vi "Library_Steering_init.vi"(8 "error in (no error)":errorcluster) -> (0 "error out":errorcluster)   [LabVIEW 2013]
uses:
  My Computer/Controls/Steering Inputs.ctl
  My Computer/Controls/Intuitive Steering.ctl
  My Computer/Controls/Servo Position.ctl
  My Computer/Controls/Fin Arrangement.ctl
  My Computer/Controls/Fin Status.ctl
  My Computer/Controls/Steering Mode.ctl
  My Computer/Controls/Individual Steering.ctl
  My Computer/Controls/IndividualSteering_f(x)_enum.ctl
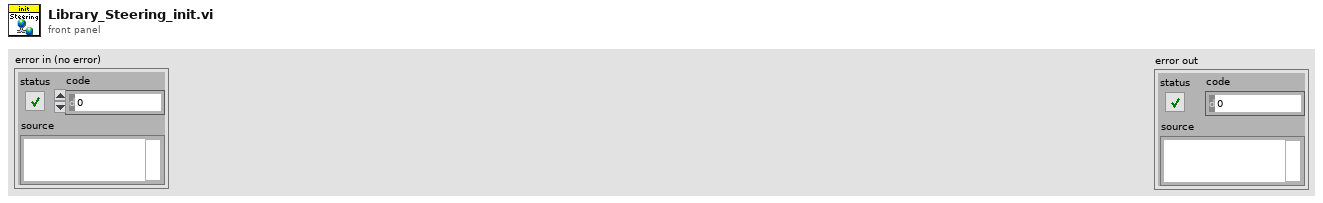
[diagram p1: front panel]
types:
  T1 = typedef "IndividualSteering_f(x)_enum.ctl" = enum16{"sin(x)", "cuttlefish sine", "cuttlefish triangle", "triangle"}
  T2 = typedef "Individual Steering.ctl" = cluster{"Fin Parameters":cluster{"Amplitude":dbl, "Phase Shift":dbl, "Zero Position":dbl}[], "Frequency\n& Direction":dbl, "General A, PS, ZP":cluster{"Amplitude":dbl, "Phase Shift":dbl, "Zero Position":dbl}}[]
  T3 = typedef "Steering Mode.ctl" = enum16{"Intuitive Steering", "Control Allocation", "Individually"}
  T4 = typedef "Intuitive Steering.ctl" = cluster{"Frequency (Hz):":dbl, "Max. Amplitude (°):":dbl, "Phase Shift (/Pi):":dbl, "Flap (°):":dbl, "Flap Saturation:":dbl}
  T5 = typedef "Fin Status.ctl" = u32[]
  T6 = typedef "Fin Arrangement.ctl" = cluster{"Fin0":u8, "Fin3":u8, "Fin1":u8, "Fin2":u8}
  T7 = typedef "Servo Position.ctl" = dbl[][]
  T8 = typedef "Steering Inputs.ctl" = cluster{"X":dbl, "Y":dbl, "Z":dbl, "phi":dbl, "theta":dbl, "psi":dbl}
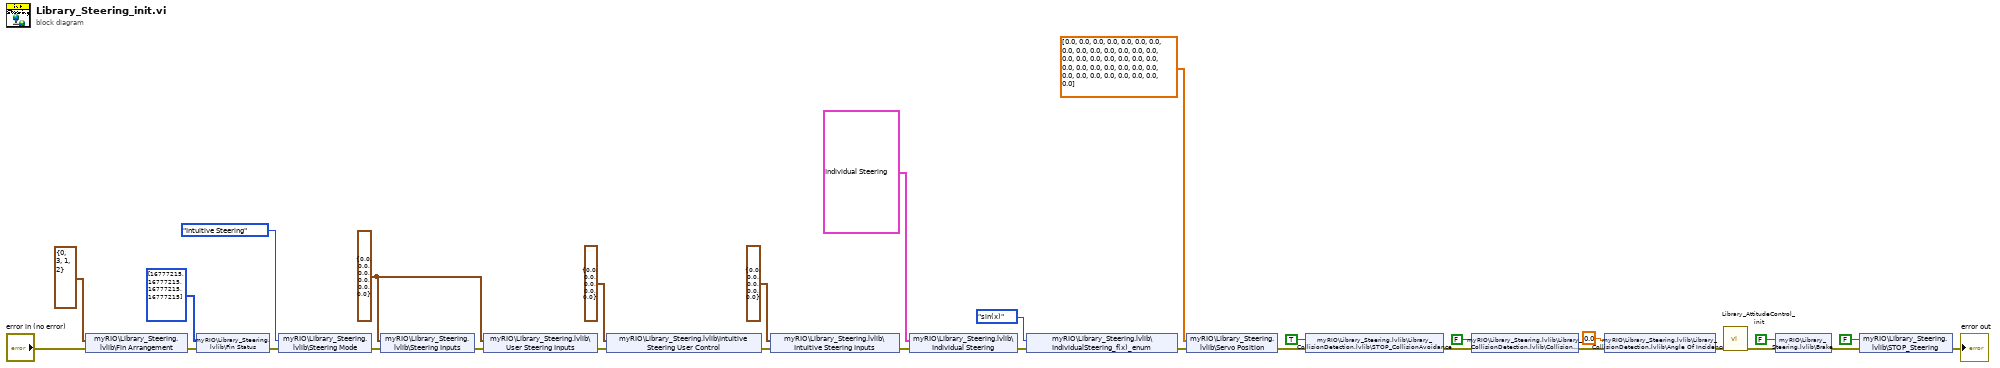
[diagram p0: block diagram]
diagram:
  w18 = T8 {"X"=0.0, "Y"=0.0, "Z"=0.0, "phi"=0.0, "theta"=0.0, "psi"=0.0} ("Steering Inputs")
  n1 = shared-variable "myRIO\\Library_Steering.lvlib\\Fin Arrangement"(T6 {"Fin0"=0, "Fin3"=3, "Fin1"=1, "Fin2"=2} ("Fin Arrangement"), error in="error in (no error)") -> (error out=w26:errorcluster)
  n2 = shared-variable "myRIO\\Library_Steering.lvlib\\Fin Status"(T5 [16777215, 16777215, 16777215, 16777215] ("Fin Status"), error in=w26) -> (error out=w25:errorcluster)
  n3 = shared-variable "myRIO\\Library_Steering.lvlib\\Steering Mode"(Steering_Mode."Intuitive Steering" ("Steering Mode"), error in=w25) -> (error out=w24:errorcluster)
  n4 = shared-variable "myRIO\\Library_Steering.lvlib\\Steering Inputs"(w18, error in=w24) -> (error out=w17:errorcluster)
  n5 = shared-variable "myRIO\\Library_Steering.lvlib\\User Steering Inputs"(w18, error in=w17) -> (error out=w16:errorcluster)
  n6 = shared-variable "myRIO\\Library_Steering.lvlib\\Intuitive Steering User Control"(T4 {"Frequency (Hz):"=0.0, "Max. Amplitude (°):"=0.0, "Phase Shift (/Pi):"=0.0, "Flap (°):"=0.0, "Flap Saturation:"=0.0} ("Intuitive Steering"), error in=w16) -> (error out=w14:errorcluster)
  n7 = shared-variable "myRIO\\Library_Steering.lvlib\\Intuitive Steering Inputs"(T4 {"Frequency (Hz):"=0.0, "Max. Amplitude (°):"=0.0, "Phase Shift (/Pi):"=0.0, "Flap (°):"=0.0, "Flap Saturation:"=0.0} ("Intuitive Steering Inputs"), error in=w14) -> (error out=w11:errorcluster)
  n8 = shared-variable "myRIO\\Library_Steering.lvlib\\Individual Steering"(T2 [{"Fin Parameters"=[{"Amplitude"=30.0, "Phase Shift"=0.25, "Zero Position"=0.0}, {"Amplitude"=30.0, "Phase Shift"=0.25, "Zero Position"=0.0}, {"Amplitude"=30.0, "Phase Shift"=0.25, "Zero Position"=0.0}, {"Amplitude"=30.0, "Phase Shift"=0.25, "Zero Position"=0.0}, {"Amplitude"=30.0, "Phase Shift"=0.25, "Zero Position"=0.0}, {"Amplitude"=30.0, "Phase Shift"=0.25, "Zero Position"=0.0}, {"Amplitude"=30.0, "Phase Shift"=0.25, "Zero Position"=0.0}, {"Amplitude"=30.0, "Phase Shift"=0.25, "Zero Position"=0.0}, {"Amplitude"=30.0, "Phase Shift"=0.25, "Zero Position"=0.0}], "Frequency\n& Direction"=1.0, "General A, PS, ZP"={"Amplitude"=30.0, "Phase Shift"=0.25, "Zero Position"=0.0}}, {"Fin Parameters"=[{"Amplitude"=30.0, "Phase Shift"=0.25, "Zero Position"=0.0}, {"Amplitude"=30.0, "Phase Shift"=0.25, "Zero Position"=0.0}, {"Amplitude"=30.0, "Phase Shift"=0.25, "Zero Position"=0.0}, {"Amplitude"=30.0, "Phase Shift"=0.25, "Zero Position"=0.0}, {"Amplitude"=30.0, "Phase Shift"=0.25, "Zero Position"=0.0}, {"Amplitude"=30.0, "Phase Shift"=0.25, "Zero Position"=0.0}, {"Amplitude"=30.0, "Phase Shift"=0.25, "Zero Position"=0.0}, {"Amplitude"=30.0, "Phase Shift"=0.25, "Zero Position"=0.0}, {"Amplitude"=30.0, "Phase Shift"=0.25, "Zero Position"=0.0}], "Frequency\n& Direction"=1.0, "General A, PS, ZP"={"Amplitude"=30.0, "Phase Shift"=0.25, "Zero Position"=0.0}}, {"Fin Parameters"=[{"Amplitude"=30.0, "Phase Shift"=0.25, "Zero Position"=0.0}, {"Amplitude"=30.0, "Phase Shift"=0.25, "Zero Position"=0.0}, {"Amplitude"=30.0, "Phase Shift"=0.25, "Zero Position"=0.0}, {"Amplitude"=30.0, "Phase Shift"=0.25, "Zero Position"=0.0}, {"Amplitude"=30.0, "Phase Shift"=0.25, "Zero Position"=0.0}, {"Amplitude"=30.0, "Phase Shift"=0.25, "Zero Position"=0.0}, {"Amplitude"=30.0, "Phase Shift"=0.25, "Zero Position"=0.0}, {"Amplitude"=30.0, "Phase Shift"=0.25, "Zero Position"=0.0}, {"Amplitude"=30.0, "Phase Shift"=0.25, "Zero Position"=0.0}], "Frequency\n& Direction"=1.0, "General A, PS, ZP"={"Amplitude"=30.0, "Phase Shift"=0.25, "Zero Position"=0.0}}, {"Fin Parameters"=[{"Amplitude"=30.0, "Phase Shift"=0.25, "Zero Position"=0.0}, {"Amplitude"=30.0, "Phase Shift"=0.25, "Zero Position"=0.0}, {"Amplitude"=30.0, "Phase Shift"=0.25, "Zero Position"=0.0}, {"Amplitude"=30.0, "Phase Shift"=0.25, "Zero Position"=0.0}, {"Amplitude"=30.0, "Phase Shift"=0.25, "Zero Position"=0.0}, {"Amplitude"=30.0, "Phase Shift"=0.25, "Zero Position"=0.0}, {"Amplitude"=30.0, "Phase Shift"=0.25, "Zero Position"=0.0}, {"Amplitude"=30.0, "Phase Shift"=0.25, "Zero Position"=0.0}, {"Amplitude"=30.0, "Phase Shift"=0.25, "Zero Position"=0.0}], "Frequency\n& Direction"=1.0, "General A, PS, ZP"={"Amplitude"=30.0, "Phase Shift"=0.25, "Zero Position"=0.0}}] ("Individual Steering"), error in=w11) -> (error out=w9:errorcluster)
  n9 = shared-variable "myRIO\\Library_Steering.lvlib\\IndividualSteering_f(x)_enum"(IndividualSteering_f(x)_enum."sin(x)" ("IndividualSteering_f(x)_enum"), error in=w9) -> (error out=w8:errorcluster)
  n10 = shared-variable "myRIO\\Library_Steering.lvlib\\Servo Position"(T7 [[0.0, 0.0, 0.0, 0.0, 0.0, 0.0, 0.0, 0.0, 0.0], [0.0, 0.0, 0.0, 0.0, 0.0, 0.0, 0.0, 0.0, 0.0], [0.0, 0.0, 0.0, 0.0, 0.0, 0.0, 0.0, 0.0, 0.0], [0.0, 0.0, 0.0, 0.0, 0.0, 0.0, 0.0, 0.0, 0.0]] ("Servos Position"), error in=w8) -> (error out=w5:errorcluster)
  n11 = shared-variable "myRIO\\Library_Steering.lvlib\\Library_CollisionDetection.lvlib\\STOP_CollisionAvoidance"(TRUE ("STOP_CollisionDetection"), error in=w5) -> (error out=w4:errorcluster)
  n12 = shared-variable "myRIO\\Library_Steering.lvlib\\Library_CollisionDetection.lvlib\\Collision Detected"(FALSE ("Collision Detected"), error in=w4) -> (error out=w2:errorcluster)
  n13 = shared-variable "myRIO\\Library_Steering.lvlib\\Library_CollisionDetection.lvlib\\Angle Of Incidence"(0.0 ("Angle Of Incidence"), error in=w2) -> (error out=w1:errorcluster)
  n14 = call "Library_AttitudeControl_init.vi"("error in (no error)"=w1) -> ("error out"=w19:errorcluster)  [unwired: 10 in]
  n15 = shared-variable "myRIO\\Library_Steering.lvlib\\Brake"(FALSE ("Check-VI_Intervention"), error in=w19) -> (error out=w21:errorcluster)
  n16 = shared-variable "myRIO\\Library_Steering.lvlib\\STOP_Steering"(FALSE ("STOP_Steering"), error in=w21) -> (error out=→"error out":errorcluster)
